vi "test_stop_and_wait.vi"() -> ()   [LabVIEW 2013]
uses:
  Classes/Flags/flag.lvclass
  global variables.vi
panel:
  in  "OK Button":bool
  in  "notifier name":string="test"
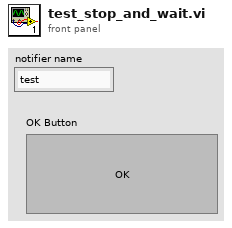
[diagram p1: front panel]
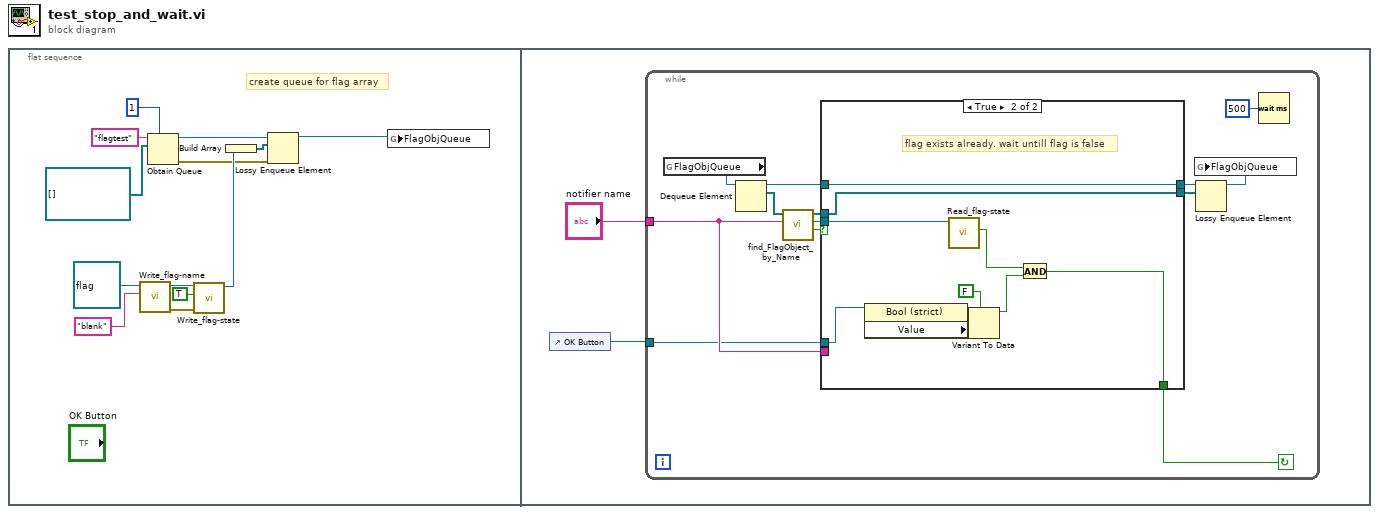
[diagram p0: block diagram]
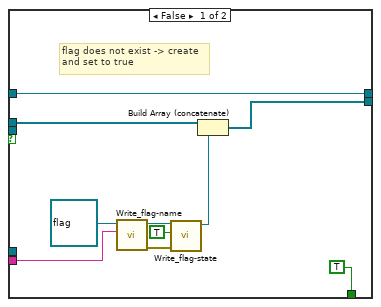
[diagram p2: hidden frame]
diagram:
  n1 = flat-sequence {
    frame #0 {
      # "create queue for flag array"
      n2 = call-dynamic "Write_flag-name.vi"("flag name"="blank", "flag in"=refnum<class "flag.lvclass"> refnum ("flag.lvclass")) -> ("error out"=w8:errorcluster, "flag out"=w9:refnum<class "flag.lvclass">)  [unwired: 8 in]
      n3 = Obtain Queue(max queue size (-1, unlimited)=1, name (unnamed)="flagtest", element data type=refnum<class "flag.lvclass">[] []) -> (queue out=w6:refnum<queue>, error out=w3:errorcluster)  [unwired: 2 in, 1 out]
      n4 = call-dynamic "Write_flag-state.vi"("error in (no error)"=w8, "flag state"=TRUE, "flag in"=w9) -> ("flag out"=w4:refnum<class "flag.lvclass">)  [unwired: 7 in, 1 out]
      n5 = Build Array(w4) -> (w5:refnum<class "flag.lvclass">[])
      n6 = Lossy Enqueue Element(queue=w6, element=w5, error in (no error)=w3) -> (queue out=w2:refnum<queue>)  [unwired: 3 out]
      n7 = global write "global variables.vi" "FlagObjQueue"(w2) -> ()
    }
    frame #1 {
      n8 = control-ref of="OK Button"() -> (w14:refnum<vi>)
      n9 = while {
        tunnel: "notifier name" -> [w24]
        tunnel: w14 -> [w21]
        stop <- w23 continue-if-true
        n10 = global read "global variables.vi" "FlagObjQueue"() -> (w28:refnum<queue>)
        n11 = Dequeue Element(queue=w28) -> (queue out=w26:refnum<queue>, element=w18:refnum<class "flag.lvclass">[])  [unwired: 2 in, 2 out]
        n12 = call "find_FlagObject_by_Name.vi"("Flag Name"=w24, "FlagObj Array"=w18) -> ("found?"=w27:bool, "found FlagObj out"=w22:refnum<class "flag.lvclass">, "FlagObj Array out"=w25:refnum<class "flag.lvclass">[])  [unwired: 6 in, 1 out]
        n13 = case shown="True" w27 {
          tunnel: w26 -> [w30 w43]
          tunnel: w25 -> [w37 w42]
          tunnel: w24 -> [w38 _]
          tunnel: [TRUE w39] -> w23
          tunnel: w22 -> [_ w48]
          tunnel: w21 -> [_ w47]
          tunnel: [w30 w43] -> w20
          tunnel: [w29 w42] -> w19
          frame False {
            # "flag does not exist -> create\nand set to true"
            n14 = call-dynamic "Write_flag-name.vi"("flag name"=w38, "flag in"=refnum<class "flag.lvclass"> refnum ("flag.lvclass")) -> ("error out"=w34:errorcluster, "flag out"=w35:refnum<class "flag.lvclass">)  [unwired: 8 in]
            n15 = call-dynamic "Write_flag-state.vi"("error in (no error)"=w34, "flag state"=TRUE, "flag in"=w35) -> ("flag out"=w32:refnum<class "flag.lvclass">)  [unwired: 7 in, 1 out]
            n16 = Build Array (concatenate)(w37, w32) -> (w29:refnum<class "flag.lvclass">[])
          }
          frame True {
            # "flag exists already. wait untill flag is false"
            n17 = property class="Bool (strict)"(reference=w47) -> (error out=w46:errorcluster, "Value"=w45:bool)  [unwired: 1 in, 1 out]
            n18 = call-dynamic "Read_flag-state.vi"("flag in"=w48) -> ("flag state"=w41:bool)  [unwired: 8 in, 2 out]
            n19 = Variant To Data(error in=w46, type=FALSE, Variant=w45) -> (data=w40:bool)  [unwired: 1 out]
            n20 = And(x=w41, y=w40) -> (x .and. y?=w39:bool)
          }
        }
        n21 = Lossy Enqueue Element(queue=w20, element=w19) -> (queue out=w17:refnum<queue>)  [unwired: 1 in, 3 out]
        n22 = global write "global variables.vi" "FlagObjQueue"(w17) -> ()
        n23 = Wait (ms)(milliseconds to wait=u32 500) -> ()  [unwired: 1 out]
      }
    }
  }
